vi "template.vi"   [LabVIEW 2018]
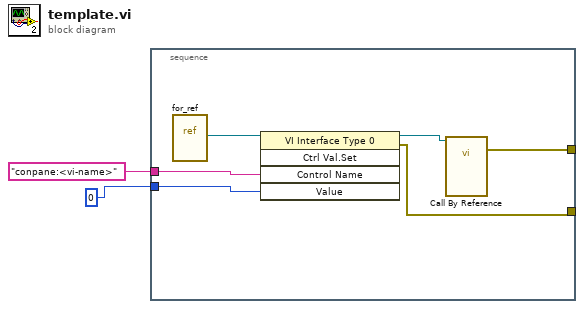
[diagram p0: block diagram]
diagram:
  n1 = stacked-sequence {
    tunnel: "conpane:<vi-name>" ("Control Name") -> [w7]
    tunnel: 0 -> [w6]
    tunnel: [w4] -> _
    tunnel: [w3] -> _
    frame #0 {
      n2 = vi-ref "for_ref.vi"() -> (w8:refnum<vi>)
      n3 = invoke class="VI Interface Type 0" method="Ctrl Val.Set"(reference=w8, "Control Name"=w7, "Value"=w6) -> (reference out=w5:refnum<vi>, error out=w3:errorcluster)  [unwired: 2 in, 3 out]
      n4 = call-by-ref "?"(reference=w5) -> (error out=w4:errorcluster)  [unwired: 2 in, 1 out]
    }
  }
